vi "trackTimerPlayground.vi"() -> ()   [LabVIEW 2017]
panel:
  out "Time has Elapsed":bool
  out "Run Time":dbl caption="Elapsed Time (s)"
  out "Error Out":errorcluster
  in  "Error In":errorcluster
  in  "Target Time to Brake":dbl=30.0 caption="Time Target (s)"
  in  "Stop SImulation VI":bool
  in  "Wheel Stripe Counter":u32
  # "Directions for simulator:\n1. Run the VI\n2. Note that the Run Time is zero until Wheel Stripe Counter is >0\n3. Set Target Time to Break (default 30 sec.)\n4. To begin the track run, increment Wheel Stripe Counter to anything greater than 0.\n5. Watch Run Time increase until it is greater than Target Time to Brake, then Time has Elapsed will turn True. NOTE: it can be changed during the run\n6. Hit Stop SImulation VI to end simulation"
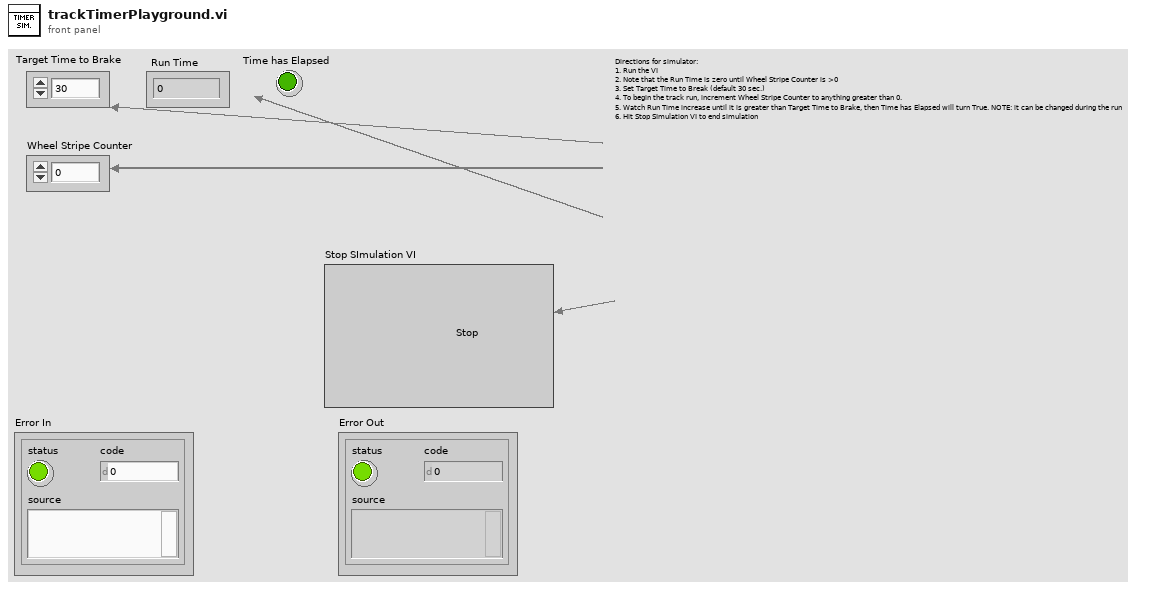
[diagram p1: front panel]
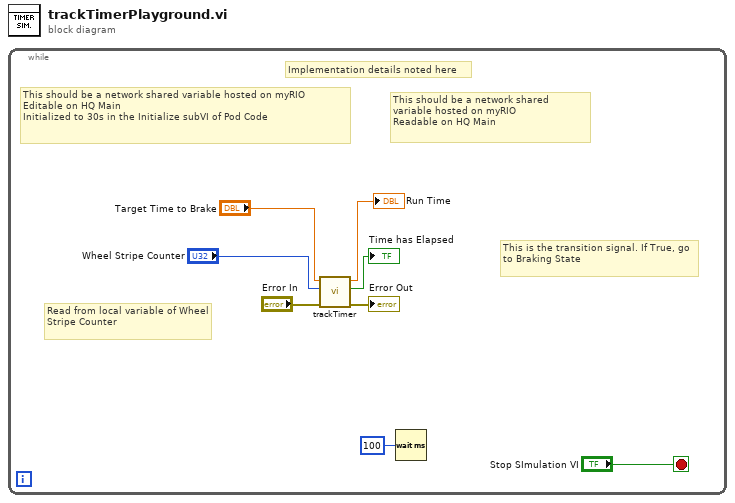
[diagram p0: block diagram]
diagram:
  n1 = while {
    stop <- "Stop SImulation VI" stop-if-true
    # "This is the transition signal. If True, go to Braking State"
    # "This should be a network shared variable hosted on myRIO\nReadable on HQ Main"
    # "Implementation details noted here"
    # "Read from local variable of Wheel Stripe Counter"
    # "This should be a network shared variable hosted on myRIO\nEditable on HQ Main\nInitialized to 30s in the Initialize subVI of Pod Code"
    n2 = call "trackTimer.vi"("error in (no error)"="Error In", "Wheel Stripe Counter"="Wheel Stripe Counter", "Time Target (s)"="Target Time to Brake") -> ("error out"=→"Error Out":errorcluster, "Time has Elapsed"=→"Time has Elapsed":bool, "Elapsed Time (s)"=→"Run Time":dbl)  [unwired: 6 in]
    n3 = Wait (ms)(milliseconds to wait=u32 100) -> ()  [unwired: 1 out]
  }
